vi "Boiler System Open.vi"(8 "error in":errorcluster) -> (0 "error out":errorcluster, 2 "Notifiers":T1, 3 "Message Queues":T2, 5 "User Event - Stop":refnum<user-event>, 7 "Stop Event Registration Refnum":refnum<event-registration>)   [LabVIEW 2022 SP3]
uses:
  Message Queue/All Message Queues.ctl
  Message Queue/Message Cluster.ctl
  Notifiers/Notifiers.ctl
  User Event - Stop/User Event - Stop.lvlib
  Message Queue/Message Queue.lvlib
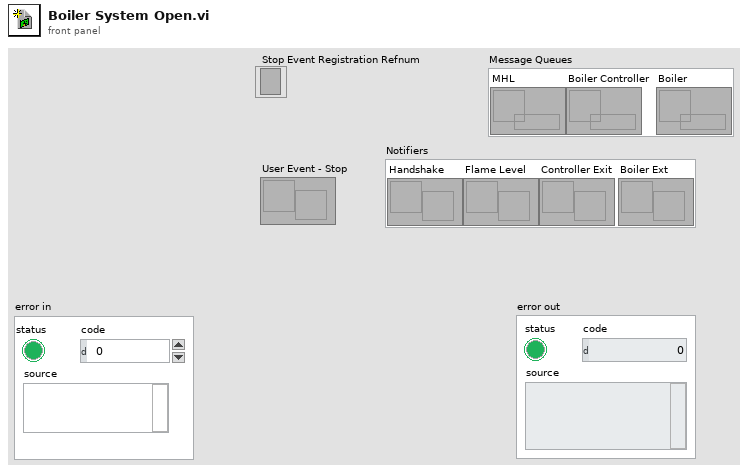
[diagram p1: front panel]
types:
  T1 = typedef "Notifiers.ctl" = cluster{"Handshake":refnum<notifier>, "Flame Level":refnum<notifier>, "Controller Exit":refnum<notifier>, "Boiler Ext":refnum<notifier>}
  T2 = typedef "Message Queue.lvlib/All Message Queues.ctl" = cluster{"MHL":refnum<queue>, "Boiler Controller":refnum<queue>, "Boiler":refnum<queue>}
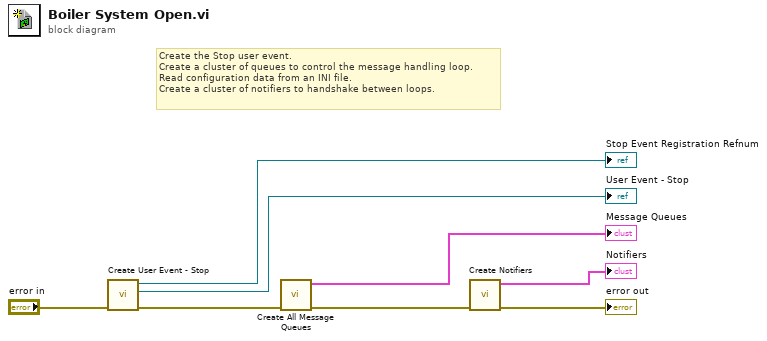
[diagram p0: block diagram]
diagram:
  # "Create the Stop user event.\nCreate a cluster of queues to control the message handling loop.\nRead configuration data from an INI file.\nCreate a cluster of notifiers to handshake between loops."
  n1 = call "Create User Event - Stop.vi"("error in"="error in") -> ("error out"=w8:errorcluster, "User Event - Stop"=→"User Event - Stop":refnum<user-event>, "Stop Event Registration Refnum"=→"Stop Event Registration Refnum":refnum<event-registration>)  [unwired: 8 in]
  n2 = call "Create All Message Queues.vi"("error in"=w8) -> ("error out"=w7:errorcluster, "Message Queues out"=→"Message Queues":T2)  [unwired: 9 in]
  n3 = call "Create Notifiers.vi"("error in"=w7) -> ("error out"=→"error out":errorcluster, "Notifiers"=→"Notifiers":T1)  [unwired: 9 in]
